vi "convert_to_DD2.vi"(11 "Array":waveform(dbl)[][](array[waveform])) -> (3 "Dynamic Data":dynamicdata(waveform))   [LabVIEW 2019]
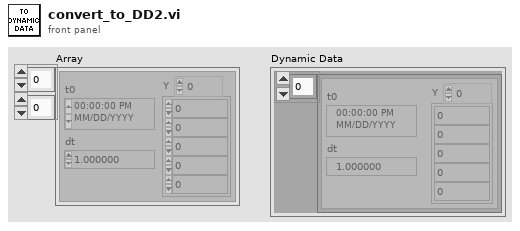
[diagram p1: front panel]
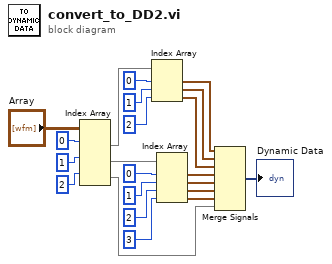
[diagram p0: block diagram]
diagram:
  n1 = Index Array(array="Array", index (row) #1=0 ("index (row)"), index (row) #2=1 ("index (row)"), index (row) #3=2 ("index (row)")) -> (element #1=w7:waveform(dbl)[], element #2=w8:waveform(dbl)[], element #3=w1:waveform(dbl)[])  [unwired: 3 in]
  n2 = Index Array(array=w7, index #1=0 ("index"), index #2=1 ("index"), index #3=2 ("index")) -> (element #1=w20:waveform(dbl), element #2=w10:waveform(dbl), element #3=w16:waveform(dbl))
  n3 = Index Array(array=w8, index #1=0 ("index"), index #2=1 ("index"), index #3=2 ("index"), index #4=3 ("index")) -> (element #1=w9:waveform(dbl), element #2=w19:waveform(dbl), element #3=w4:waveform(dbl), element #4=w3:waveform(dbl))
  n4 = Merge Signals(w20, w10, w16, w9, w19, w4, w3, w1) -> (→"Dynamic Data":dynamicdata)
